vi "Obtain I2C Message Buffer.vi"(8 "error in (no error)":errorcluster, 9 "Create (F)":bool, 10 "Msgs per Txn Queue Size (10k)":i32=10000 format="%.0p", 11 "Message Buffer Size (100k)":i32=100000 format="%.0p") -> (0 "error out":errorcluster, 2 "Msgs per Txn Queue":refnum<queue>, 3 "I2C Message Queue":refnum<queue>)   [LabVIEW 2025, in "I2C Bus Monitor.lvclass"]
uses:
  I2C Bus Monitor.lvclass
  I2C Bus Monitor.lvclass/I2C Bus Monitor.ctl
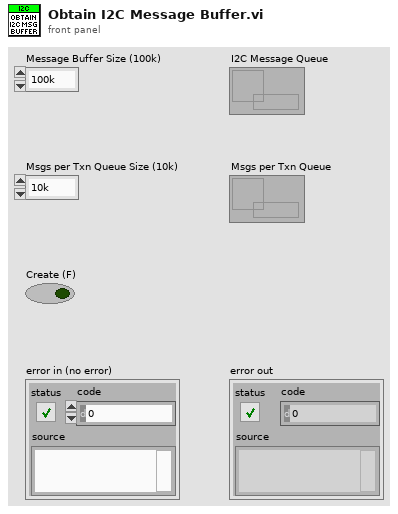
[diagram p1: front panel]
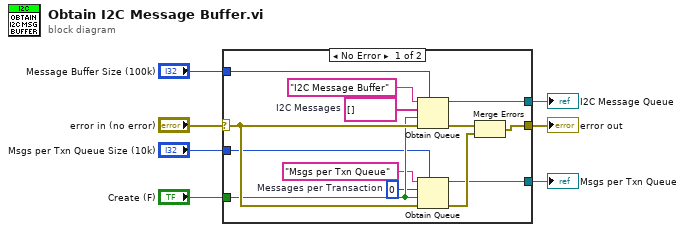
[diagram p0: block diagram]
diagram:
  n1 = case shown="No Error" "error in (no error)" {
    selector: "error in (no error)" -> [w20 w21]
    tunnel: "Create (F)" -> [w19 _]
    tunnel: "Msgs per Txn Queue Size (10k)" -> [w15 _]
    tunnel: "Message Buffer Size (100k)" -> [w14 _]
    tunnel: [w11 _] -> w3
    tunnel: [w10 _] -> w2
    tunnel: [w9 w21] -> w1
    frame No Error {
      w17 = 0  # Messages per Transaction
      w13 = string[] []  # I2C Messages
      n2 = Obtain Queue(max queue size (-1, unlimited)=w14, name (unnamed)="I2C Message Buffer", element data type=w13, create if not found? (T)=w19, error in (no error)=w20) -> (queue out=w11:refnum<queue>, error out=w8:errorcluster)  [unwired: 1 out]
      n3 = Obtain Queue(max queue size (-1, unlimited)=w15, name (unnamed)="Msgs per Txn Queue", element data type=w17, create if not found? (T)=w19, error in (no error)=w20) -> (queue out=w10:refnum<queue>, error out=w18:errorcluster)  [unwired: 1 out]
      n4 = Merge Errors(w8, w18) -> (w9:errorcluster)
    }
    frame Error {
    }
  }
  "error out" <- w1
  "I2C Message Queue" <- w3
  "Msgs per Txn Queue" <- w2
